vi "Z complex to components.vi"(6 "Angle unit":enum16{"Radians", "Degrees"}(ring), 8 "Error In":errorcluster, 9 "Z (cplx)":T3 {"Z" format="%#_4g"}) -> (0 "Error Out":errorcluster, 1 "Z unpacked":T2)   [LabVIEW 2016]
uses:
  Trace (cplx).ctl
  Trace (dbl).ctl
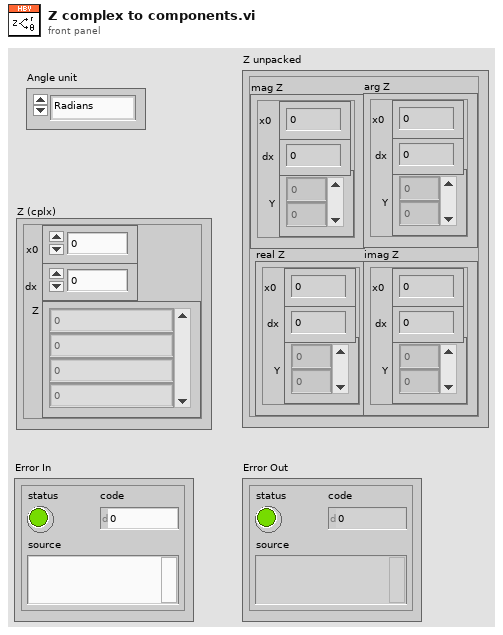
[diagram p1: front panel]
types:
  T1 = typedef "Trace (dbl).ctl" = cluster{"x0 ":dbl, "dx":dbl, "Y":dbl[]}
  T2 = cluster{"mag Z":T1, "arg Z":T1, "real Z":T1, "imag Z":T1}
  T3 = typedef "Trace (cplx).ctl" = cluster{"x0":dbl, "dx":dbl, "Z":cdb[]}
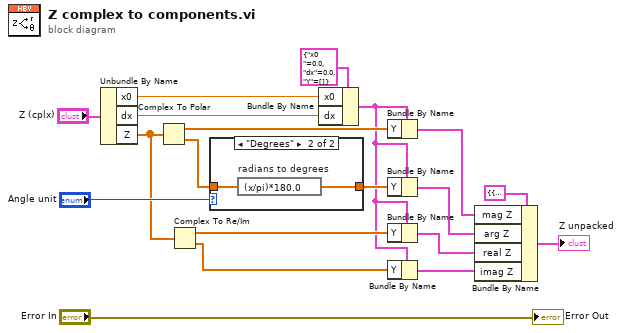
[diagram p0: block diagram]
diagram:
  n1 = Unbundle By Name("Z (cplx)") -> ("x0"=w13:dbl, "dx"=w12:dbl, "Z"=w1:cdb[])
  n2 = Complex To Polar(r * e^(i*theta)=w1) -> (r=w17:dbl[], theta=w16:dbl[])
  n3 = Complex To Re/Im(x + iy=w1) -> (x=w6:dbl[], y=w5:dbl[])
  n4 = case shown="\"Degrees\"" "Angle unit" {
    tunnel: [w20 w22] -> w19
    tunnel: w16 -> [w20 w21]
    frame "Radians", Default {
    }
    frame "Degrees" {
      n5 = expression code="(x/pi)*180.0" "radians to degrees"(w21) -> (w22:dbl[])
    }
  }
  n6 = Bundle By Name(cluster=T1 {"x0 "=0.0, "dx"=0.0, "Y"=[]} ("Spectrum"), "x0"=w13, "dx"=w12) -> (w3:T1)
  n7 = Bundle By Name(cluster=w3, "Y"=w17) -> (w9:T1)
  n8 = Bundle By Name(cluster=w3, "Y"=w19) -> (w8:T1)
  n9 = Bundle By Name(cluster=w3, "Y"=w6) -> (w4:T1)
  n10 = Bundle By Name(cluster=w3, "Y"=w5) -> (w2:T1)
  n11 = Bundle By Name(cluster=T2 {"mag Z"={"x0 "=0.0, "dx"=0.0, "Y"=[]}, "arg Z"={"x0 "=0.0, "dx"=0.0, "Y"=[]}, "real Z"={"x0 "=0.0, "dx"=0.0, "Y"=[]}, "imag Z"={"x0 "=0.0, "dx"=0.0, "Y"=[]}} ("Z unpacked 2"), "mag Z"=w9, "arg Z"=w8, "real Z"=w4, "imag Z"=w2) -> (→"Z unpacked":T2)
  "Error Out" <- "Error In"
